vi "EXAMPLE.vi"() -> ()   [LabVIEW 2017, in "VIs to Interface LabVIEW and MySQL dotNET Connector.lvlib"]
uses:
  VIs to Interface LabVIEW and MySQL dotNET Connector.lvlib
  Controls/Database Command.ctl
  Controls/Database Connection Data.ctl
panel:
  in  "?":T1={"Server"="127.0.0.1", "Port"=3306, "UserID"="root", "Password"="password", "Database"="database"}
  out "SQL Command Echo":string
  in  "Database Command":T2=enum."Select All"
  in  "Query":bool
  in  "SQL Text Command":string
  in  "Table":string="table"
  in  "Column List":string[](array[string])
  in  "Values":string[](array[string])
  in  "Condition":string
  out "Data Returned By Query":string[][](array[string])
  out "error out":errorcluster
  # "Used for Update and Insert Commands"
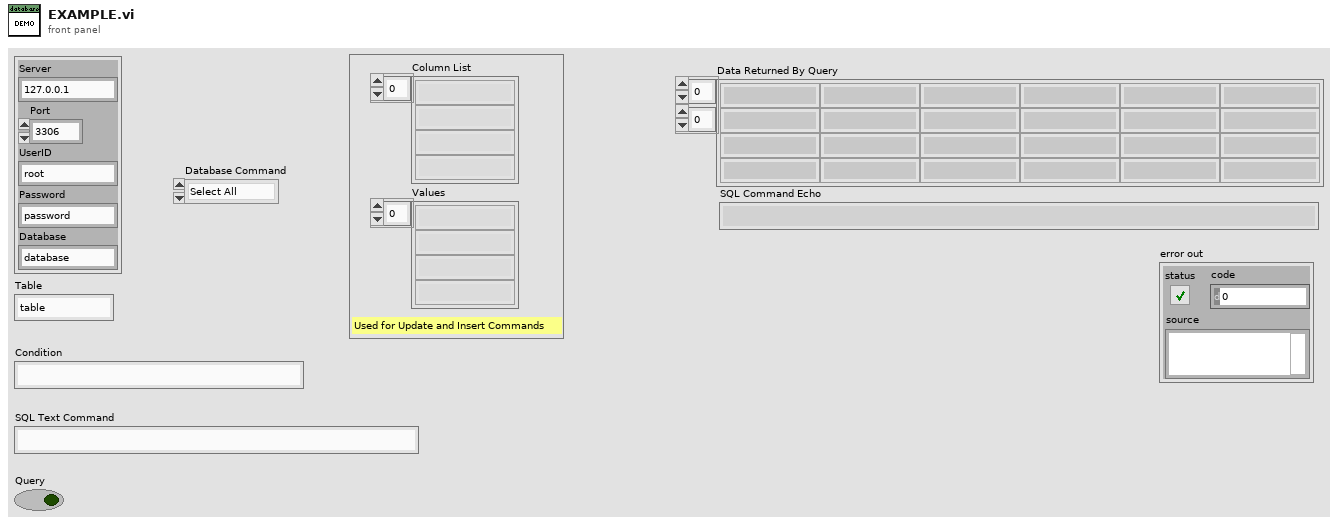
[diagram p1: front panel]
types:
  T1 = typedef "VIs to Interface LabVIEW and MySQL dotNET Connector.lvlib/Database Connection Data.ctl" = cluster{"Server":string, "Port":u32, "UserID":string, "Password":string, "Database":string}
  T2 = typedef "VIs to Interface LabVIEW and MySQL dotNET Connector.lvlib/Database Command.ctl" = enum16{"Insert", "Update", "Select All", "Delete Entry", "Drop Table", "SQL Command", "Select", "Get Column Info", "Select Column"}
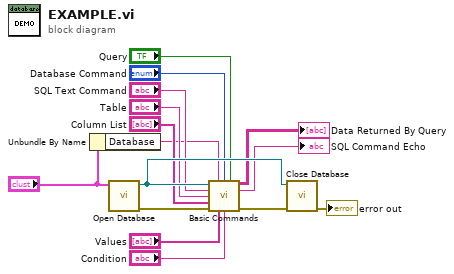
[diagram p0: block diagram]
diagram:
  n1 = Unbundle By Name("?") -> ("Database"=w1:string)
  n2 = call "Open Database.vi"(11:"?") -> ("error out"=w10:errorcluster, ".Net dbase ref"=w14:refnum<k24>)  [unwired: 9 in]
  n3 = call "Basic Commands.vi"(".NET Refnum in"=w14, "Database"=w1, "Database Command"="Database Command", "Query"="Query", "SQL Command"="SQL Text Command", "Table"="Table", "Column List"="Column List", "error in (no error)"=w10, "Values"="Values", "Condition"="Condition") -> ("Data Array"=→"Data Returned By Query":string[][], "SQL Command out"=→"SQL Command Echo":string, "error out"=w15:errorcluster)  [unwired: 3 in]
  n4 = call "Close Database.vi"("error in (no error)"=w15, ".NET Refnum in"=w14) -> ("error out"=→"error out":errorcluster)  [unwired: 9 in]
